vi "Path_Test2020_TankRobot_ScanIndex_CreateFile.vi"() -> ()   [LabVIEW 2019]
uses:
  Pathfinder-Lib/VIs/Waypoint.ctl
  <vilib>/Rock Robotics/WPI/DriverStation/WPI_DriverStationRobotMode2.ctl
  Pathfinder-Lib/VIs/Wheel_Ctrl_Path_Element.ctl
  Pathfinder-Lib/VIs/Wheel_Ctrl_Path.ctl
  Pathfinder-Lib/Pathfinder.lvlib
  Robot Global Data.vi
  <vilib>/Rock Robotics/SystemInterfaces/AI/FPGA_AIGyroChannel.ctl
  <vilib>/Rock Robotics/Network Tables/NT Write Number.vi
  <vilib>/Rock Robotics/WPI/Counter/WPI_CounterDigitalInputToDigitalSource.vi
  <vilib>/Rock Robotics/SystemInterfaces/DIO/FPGA_DIOChannel.ctl
  <vilib>/Rock Robotics/WPI/Encoder/WPI_EncoderType.ctl
  <vilib>/Rock Robotics/Network Tables/NT Write Numeric Array.vi
  <vilib>/addons/control/pid/NI_PID_pid.lvlib
  <vilib>/Rock Robotics/SystemInterfaces/DIO/FPGA_DIOPWMChannel.ctl
  <vilib>/Rock Robotics/WPI/SafetyOutput/WPI_SafetyOutputConfigMenu.ctl
  Secret_Control_Library_Protected/Secret_Control_Library_Protected.lvlib
  <vilib>/addons/control/pid/pid.llb/PID (DBL).vi
  <vilib>/Rock Robotics/WPI/Gyro/WPI_GyroAnalogOpen.vi
  <vilib>/Rock Robotics/WPI/RobotDrive/WPI_RobotDriveOpen2MotorWithTalon.vi
panel:
  in  "Tab Control 3":enum32{"Robot Data", "Path Definition"}(tab)
  in  "Real max\n speed":dbl=84.0
  in  "wheelbase_width":dbl=20.866
  in  "max_jerk":dbl=120.0
  in  "max_acceleration":dbl=65.0
  in  "max_velocity":dbl=70.0
  in  "?":T1[](array[typedef])=[{"x"=15.0, "y"=105.0, "angle"=0.0}, {"x"=35.0, "y"=105.0, "angle"=0.0}, {"x"=210.0, "y"=32.0, "angle"=0.0}, {"x"=230.0, "y"=32.0, "angle"=0.0}, {"x"=455.0, "y"=32.0, "angle"=0.0}, {"x"=625.0, "y"=98.0, "angle"=0.0}]
  in  "Path Results\ndT":dbl=0.02 format="%7.3f"
  in  "sample_count":i32=100000
  out "Path calculation error":errorcluster
  in  "Calculate\nPath":bool
  out "Complete,\nReady to \nExecute":bool
  out "Path \nSpeed > \nMax":bool
  in  "Rev\nDirection":bool
  in  "Tab Control 2":enum32{"Create File", "Robot Execution"}(tab)
  in  "Include Step":bool=TRUE
  in  "End Path CMD":i32=64
  in  "Cont Path CMD":i32=62
  in  "Start Path CMD":i32=60
  in  "Starting Step":i32
  in  "Command List Path Comment":string
  in  "Command List File Name":path
  in  "CreateCmdList":bool
  in  "Ramsete ?":bool=TRUE
  out "Robot Mode":T2
  out "Distance Error":dbl[](array[numeric]) format="%14.2f"
  out "Heading Error":dbl format="%14.2f"
  in  "Use Gyro\nCompensation":bool=TRUE
  out "Distance":dbl[](array[numeric]) format="%19.2f"
  in  "Gyro Comp PID gains":T3={"proportional gain (Kc)"=0.065, "integral time (Ti, min)"=0.004, "derivative time (Td, min)"=0.0} {"derivative time (Td, min)" format="%.4f"; "integral time (Ti, min)" format="%.4f"; "proportional gain (Kc)" format="%.4f"}
  out "Heading":dbl format="%18.2f"
  out "Gyro Comp":dbl format="%18.2f"
  out "Heading Demand":dbl format="%18.2f"
  in  "Execute\nPath":bool
  out "Robot\nExecuting":bool
  out "Path Distance":dbl[](array[numeric]) format="%19.2f"
  in  "Stop\nProgram":bool
  in  "Tab Control":T4(tab)
  out "Position":cluster{dbl[], dbl[]}[](graph)
  out "Path":T5(graph)
  out "Size":i32
  out "Robot Path Data":T6[](array[typedef]) {"D Time" format="%13.3f"; "Angle" format="%13.3f"; "R dist" format="%13.3f"; "L dist" format="%13.3f"; "R spd" format="%13.3f"; "L spd" format="%13.3f"; "T Time" format="%13.3f"}
  out "Wheel dmd":T7(graph)
  out "Gyro Cht":cluster{"GyroContinuous":dbl, "Angle":dbl}(graph)
  out "Err Chart":cluster{dbl, dbl, dbl}(graph)
  # "ROBOT DATA"
  # "INCHES/SEC"
  # "INCHES/SEC"
  # "INCHES/SEC^2"
  # "?? INCHES/SEC^3"
  # "Simulated robot is 20.866"
  # "INCHES"
  # "PATH DEFINITION"
  # "SEC"
  # "ROBOT EXECUTION\n(disabled...)"
  # "Instructions:\nThis should create a path, show the data on the various tabs and optionally write the motor demands and expected results to a file for use on a a robot..\n1) Enter robot data on Robot Data Tab\n2) Define your path definitions.\n3) Define the time increment.  0.020 is chosen since that matches the normal loop time.\n4) Press calculate path.  If a good path was calculated it will be displayed on the Tank Data tab, and the Ready to Execute will indicate execution can begin.\nThe path can be recalculated many times before selecting execute.\n\nTo write to a file.\n5) Select the file name\n6) This example uses \"steps\", sequential numbers for inclusion into a list based autonomous routine.  Including the step number if optional.\n7) This uses command numbers to indicate first, last, and intermediate steps.  This allows some simplification of the execution routine.  It\nalso allows the path to be executed backwards if desired.  The command numbers are changeable.\n8) Press \"Create Command List\".\n\nNotes:\n- PC robot simulataion is disabled in this program.  The code is still there if you want to restore it and try it out.  Use one of the other test programs \nto simulate the path on a PC.\n- The path generation logic doesn't account distribution of speed to the left and right wheels.  As a result the maximum speed can be exceeded.\nIf this happens, but Path Speed > Max light will light and Ready to Execute will not light.  Lower the maximum speed in the Robot Data tab\nand recalulate the path.\n- 2019 playing field size - width: 26 ft 11.25 In = 323.25 in , length: 52 ft 5.25 in = 629.25 in  (I didn't verify this for the 2020 version.)"
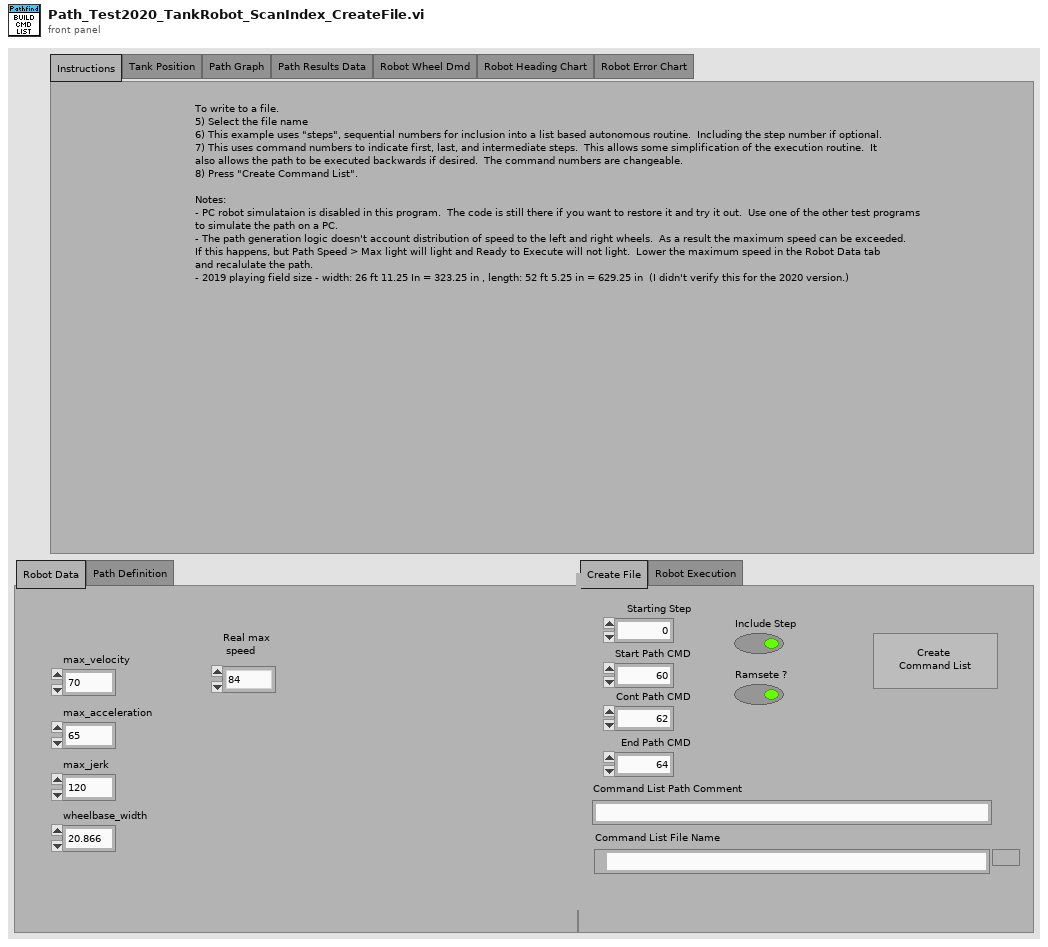
[diagram p1: front panel]
types:
  T1 = typedef "Pathfinder.lvlib/Waypoint.ctl" = cluster{"x":dbl, "y":dbl, "angle":dbl}
  T2 = typedef "WPI_DriverStationRobotMode2.ctl" = enum16{"Autonomous Disabled", "Autonomous Enabled", "Teleop Disabled", "Teleop Enabled", "Disconnected", "Finish", "Test Disabled", "Test Enabled", "Emergency Stopped"}
  T3 = cluster{"proportional gain (Kc)":dbl, "integral time (Ti, min)":dbl, "derivative time (Td, min)":dbl}
  T4 = enum32{"Instructions", "Tank Position", "Path Graph", "Path Results Data", "Robot Wheel Dmd", "Robot Heading Chart", "Robot Error Chart"}
  T5 = cluster{"position":dbl, "velocity":dbl, "acceleration":dbl, "jerk":dbl, "heading":dbl}[]
  T6 = typedef "Pathfinder.lvlib/Wheel_Ctrl_Path_Element.ctl" = cluster{"T Time":dbl, "L spd":dbl, "R spd":dbl, "L dist":dbl, "R dist":dbl, "Angle":dbl, "D Time":dbl}
  T7 = cluster{"Output":dbl, "Output":dbl, "output":dbl}
  T8 = typedef "Pathfinder.lvlib/Wheel_Ctrl_Path.ctl" = cluster{"Wheel_Ctrl_Elements":T6[], "NumberOfElements":u32, "DeltaMillseconds":i32}
  T9 = typedef "Pathfinder.lvlib/Segment.ctl" = cluster{"dt":dbl, "x":dbl, "y":dbl, "position":dbl, "velocity":dbl, "acceleration":dbl, "jerk":dbl, "heading":dbl}
  T10 = cluster{"position":dbl, "velocity":dbl, "acceleration":dbl, "jerk":dbl, "heading":dbl}
  T11 = typedef "WPI_SafetyOutputConfigMenu.ctl" = enum16{"Enable", "Disable"}
  T12 = typedef "WPI_EncoderType.ctl" = enum16{"1x", "2x", "4x"}
  T13 = typedef "FPGA_AIGyroChannel.ctl" = enum8{"AI 0", "AI 1", "Invalid"}
  T14 = enum32{"Instructions", "Robot Data", "Tank Position", "Path Graph", "Path Results Data", "Robot Wheel Dmd", "Robot Heading Chart", "Robot Error Chart"}
  T15 = typedef "FPGA_DIOPWMChannel.ctl" = enum8{"PWM 0", "PWM 1", "PWM 2", "PWM 3", "PWM 4", "PWM 5", "PWM 6", "PWM 7", "PWM 8", "PWM 9", "PWM MXP 0", "PWM MXP 1", "PWM MXP 2", "PWM MXP 3", "PWM MXP 4", "PWM MXP 5", "PWM MXP 6", "PWM MXP 7", "PWM MXP 8", "PWM MXP 9", "Invalid"}
  T16 = typedef "FPGA_DIOChannel.ctl" = enum8{"DIO 0", "DIO 1", "DIO 2", "DIO 3", "DIO 4", "DIO 5", "DIO 6", "DIO 7", "DIO 8", "DIO 9", "DIO MXP 0", "DIO MXP 1", "DIO MXP 2", "DIO MXP 3", "DIO MXP 4", "DIO MXP 5", "DIO MXP 6", "DIO MXP 7", "DIO MXP 8", "DIO MXP 9", "DIO MXP 10", "DIO MXP 11", "DIO MXP 12", "DIO MXP 13", "DIO MXP 14", "DIO MXP 15", "SPI Port CS1", "SPI Port CS2", "SPI Port CS3", "SPI Port MISO", "SPI Port MOSI", "Invalid"}
  T17 = typedef "WPI_RobotDriveDevRef.ctl" = cluster{"DevStatus":errorcluster, "Motors[]":T18[], "Square Inputs":bool, "Max Output":dbl}
  T18 = typedef "WPI_MotorControlDeviceRef.ctl" = cluster{"DeviceStatus":errorcluster, "Type":T19, "PWM":cluster{"PWM Channel":T15, "DeadBand":T20}, "CAN":cluster{"Device Number":u8, "SetOutput VI Ref":variant, "GetOutput VI Ref":variant, "Enable VI Ref":variant, "Disable VI Ref":variant, "Data":variant}, "Invert":bool, "DIO PWM":cluster{"PWM \"Enable\" Channel":T15, "DIOChannel":T16, "PWM Rate":dbl}}
  T19 = typedef "WPI_MotorControlType.ctl" = enum16{"PWM", "CAN", "DIO PWM"}
  T20 = typedef "WPI_PWMDeadband.ctl" = cluster{"Name":string, "maxPositivePwm":i32, "minPositivePwm":i32, "centerPwm":i32, "maxNegativePwm":i32, "minNegativePwm":i32, "angularRange":u16}
  T21 = typedef "WPI_DigitalInputDevRef.ctl" = cluster{"DevStatus":errorcluster, "DIO Channel":T16}
  T22 = typedef "FPGA_CounterEncoderSourceConvertionLVSourceType.ctl" = cluster{"DevStatus":errorcluster, "AnalogTriggerMode?":bool, "DigitalMode":cluster{"DIO Channel":T23}, "AnalogTriggerMode":cluster{"AnalogTriggerIndex":T24, "OutputType":T25}}
  T23 = typedef "FPGA_DIODigitalSourceChannel.ctl" = enum8{"DIO 0", "DIO 1", "DIO 2", "DIO 3", "DIO 4", "DIO 5", "DIO 6", "DIO 7", "DIO 8", "DIO 9", "DIO MXP 0", "DIO MXP 1", "DIO MXP 2", "DIO MXP 3", "DIO MXP 4", "DIO MXP 5", "DIO MXP 6", "DIO MXP 7", "DIO MXP 8", "DIO MXP 9", "DIO MXP 10", "DIO MXP 11", "DIO MXP 12", "DIO MXP 13", "DIO MXP 14", "DIO MXP 15", "SPI Port CS1", "SPI Port CS2", "SPI Port CS3", "SPI Port MISO", "SPI Port MOSI", "Disabled"}
  T24 = typedef "FPGA_AnalogTriggerIndex.ctl" = enum8{"Trig 0", "Trig 1", "Trig 2", "Trig 3", "Trig 4", "Trig 5", "Trig 6", "Trig 7", "Invalid"}
  T25 = typedef "FPGA_AnalogTriggerOutType.ctl" = enum16{"InWindow", "TriggerState", "Rising", "Falling"}
  T26 = typedef "WPI_EncoderDevRef.ctl" = cluster{"DevStatus":errorcluster, "EncoderIndex":T27, "CounterIndex":T28, "DistancePerCount":dbl, "Decoding Type":T12}
  T27 = typedef "FPGA_EncoderIdx.ctl" = enum8{"Enc 0", "Enc 1", "Enc 2", "Enc 3", "Enc 4", "Enc 5", "Enc 6", "Enc 7", "Invalid"}
  T28 = typedef "FPGA_CounterCtrSystemIndex.ctl" = enum8{"Ctr 0", "Ctr 1", "Ctr 2", "Ctr 3", "Ctr 4", "Ctr 5", "Ctr 6", "Ctr 7", "Invalid"}
  T29 = typedef "WPI_GyroDevRef.ctl" = cluster{"DevStatus":errorcluster, "Analog Channel":T30, "Gain (VoltsPerDegree/Second)":dbl, "Gyro Type":enum16{"Analog", "XRS450"}, "Handle":i32, "SPI Bus":T31, "Device Found":bool, "Sample Rate":dbl, "Calibrate On Open":bool, "Offset":dbl}
  T30 = typedef "FPGA_AIChannel.ctl" = enum8{"AI 0", "AI 1", "AI 2", "AI 3", "AI MXP 0", "AI MXP 1", "AI MXP 2", "AI MXP 3", "Invalid"}
  T31 = typedef "spi_bus.ctl" = enum16{"SPI On-Board, CS0", "SPI On-Board, CS1", "SPI On-Board, CS2", "SPI On-Board, CS3", "SPI MXP", "Invalid"}
  T32 = cluster{"GyroContinuous":dbl, "GyroContinuous":dbl}
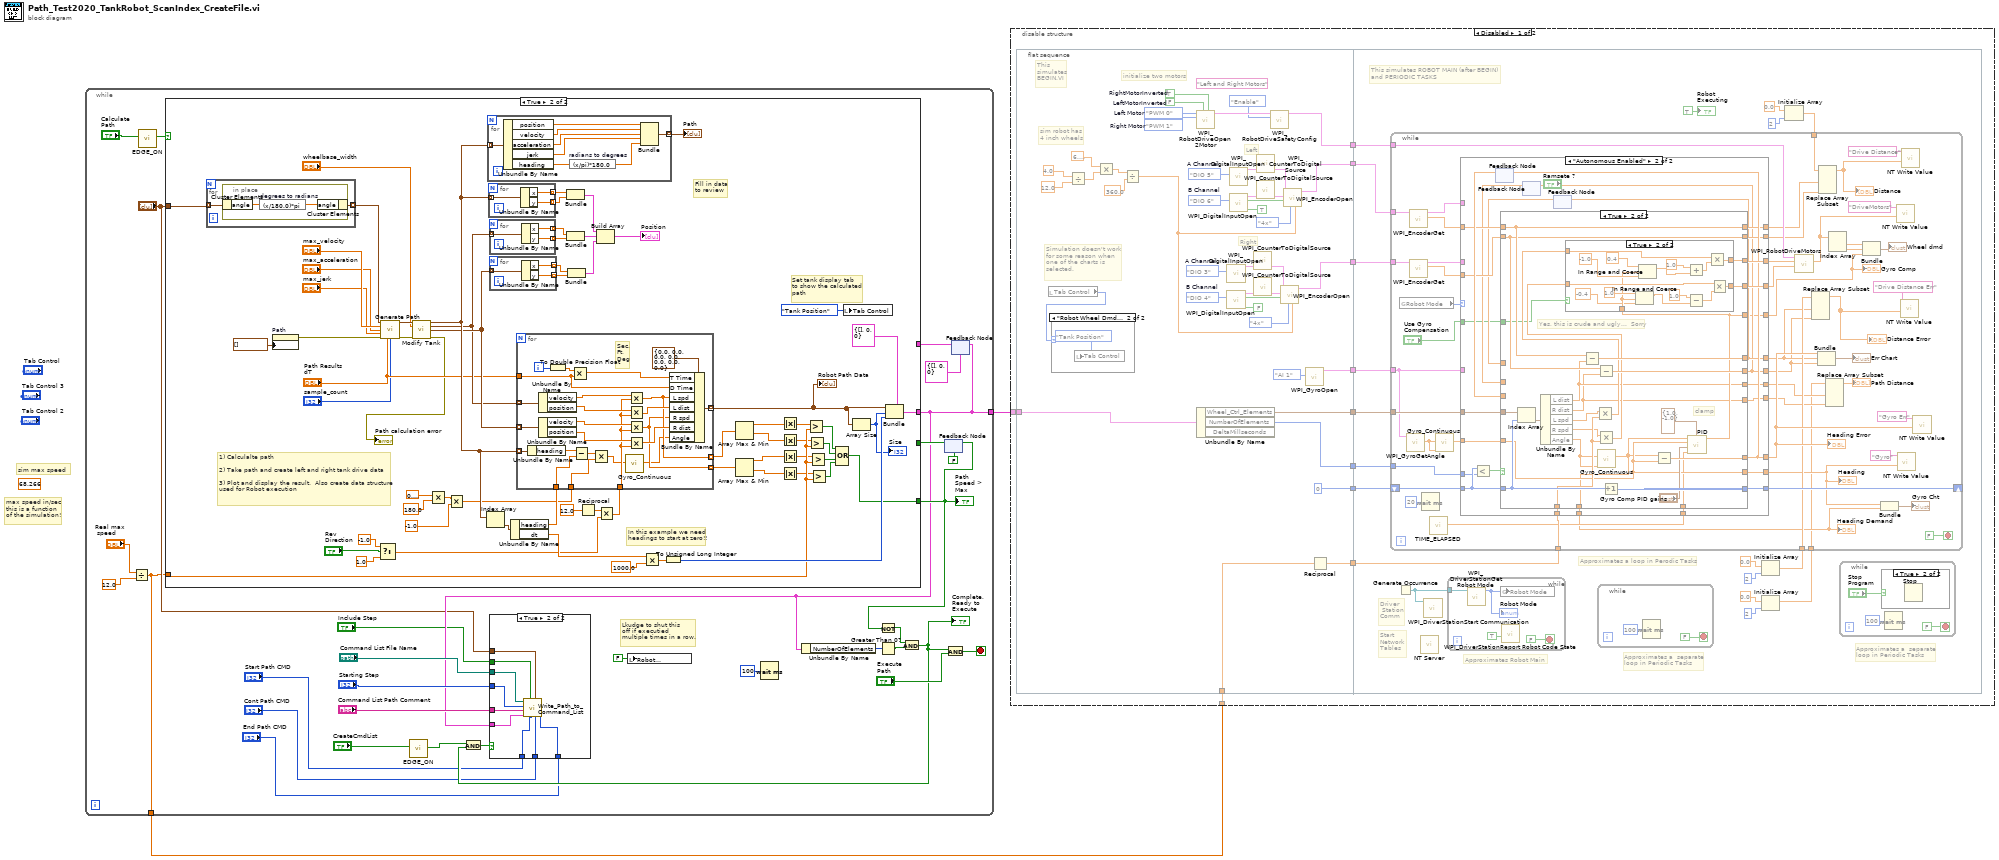
[diagram p0: block diagram]
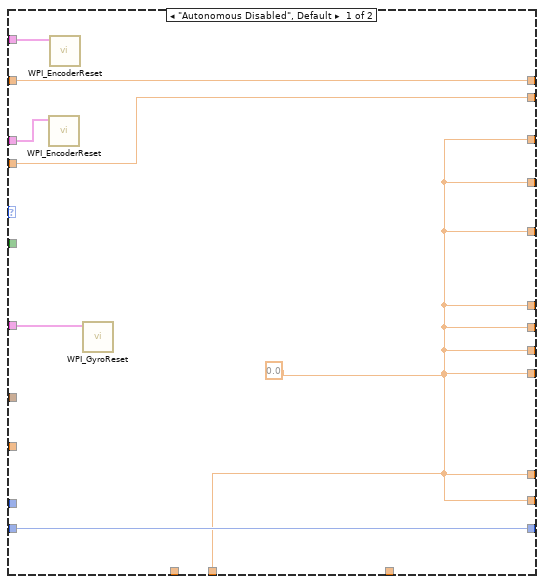
[diagram p4: hidden frame]
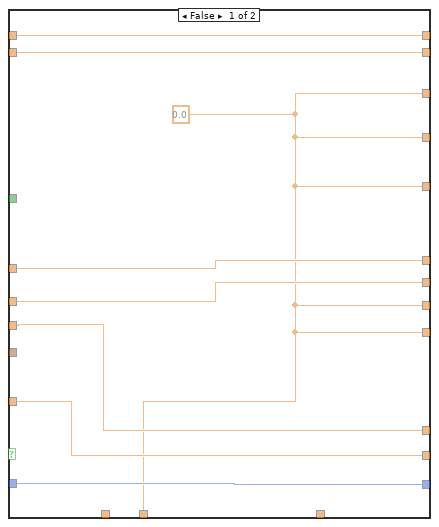
[diagram p5: hidden frame]
diagram:
  (unwired) 68.266 ("x")
  # "sim max speed"
  # "max speed in/sec\nthis is a function\nof the simulation!"
  n1 = while {
    tunnel: [w11] -> w2
    tunnel: [w3] -> w1
    stop <- w25 stop-if-true
    # "Lkudge to shut this\noff if executied\nmultiple times in a row."
    n2 = Divide(x="Real max\n speed", y=12.0) -> (x/y=w3:dbl)
    n3 = call "EDGE_ON.vi"("INPUT"="Calculate\nPath") -> ("EDGE ON"=w30:bool)  [unwired: 10 in]
    n4 = call "EDGE_ON.vi"("INPUT"="CreateCmdList") -> ("EDGE ON"=w13:bool)  [unwired: 10 in]
    n5 = local write "Robot\nExecuting"(FALSE ("Robot\nExecuting")) -> ()
    n6 = Wait (ms)(milliseconds to wait=u32 100) -> ()  [unwired: 1 out]
    n7 = feedback #1(FALSE) -> (w22:bool)
    n8 = feedback #2(T8 {"Wheel_Ctrl_Elements"=[], "NumberOfElements"=0, "DeltaMillseconds"=0} ("Wheel_Ctrl_Elements")) -> (w28:T8)
    n9 = case shown="True" w30 {
      tunnel: [w43 w71] -> w11
      tunnel: w28 -> [w43 _]
      tunnel: w3 -> [_ w69]
      tunnel: [w42 w60] -> w19
      tunnel: w22 -> [w42 _]
      tunnel: "?" -> [_ w50]
      frame False {
      }
      frame True {
        # "Set tank display tab\nto show the calculated\npath"
        # "Fill in data\nto review"
        # "1) Calculalte path\n\n2) Take path and create left and right tank drive data\n\n3) Plot and display the result.  Also create data structure\nused for Robot execution"
        # "In this example we need\nheadings to start at zero!!"
        n10 = for {
          tunnel: w50 -> [w135] mode=indexing
          tunnel: [w134] -> w97 mode=indexing
          n11 = in-place {
            n12 = in-place-cluster #3(w135) -> ("angle"=w137:dbl)
            n13 = expression code="(x/180.0)*pi" "degrees to radians"(w137) -> (w136:dbl)
            n14 = in-place-cluster #3("angle"=w136) -> (w134:T1)
          }
        }
        n15 = property on="Path" class="WFChart (strict)"("History Data"=T5 []) -> (error out=w98:errorcluster)  [unwired: 2 in, 1 out]
        n16 = Select(t=-1.0, s="Rev\nDirection", f=1.0) -> (s? t:f=w44:dbl)
        n17 = call "Generate Path.vi"("path"=w97, "max_velocity"="max_velocity", "max_acceleration"="max_acceleration", "max_jerk"="max_jerk", "error in"=w98, "dt (.001)"="Path Results\ndT", "sample_count (100000)"="sample_count") -> ("Segments"=w99:T9[], "error out"=w86:errorcluster)  [unwired: 7 in]
        n18 = call "Modify Tank.vi"("Original"=w99, "wheelbase_width"="wheelbase_width", "error in"=w86) -> ("original"=w107:T9[], "left"=w103:T9[], "right"=w104:T9[], "error out"=→"Path calculation error":errorcluster)  [unwired: 9 in]
        n19 = Multiply(x=0.3183098861837907, y=180.0) -> (x*y=w106:dbl)
        n20 = Multiply(x=w106, y=-1.0) -> (x*y=w52:dbl)
        n21 = Index Array(array=w107) -> (element=w108:T9)  [unwired: 1 in]
        n22 = for {
          tunnel: w107 -> [w154] mode=indexing
          tunnel: [w148] -> w101 mode=indexing
          n23 = Unbundle By Name(w154) -> ("position"=w153:dbl, "velocity"=w152:dbl, "acceleration"=w151:dbl, "jerk"=w150:dbl, "heading"=w149:dbl)
          n24 = expression code="(x/pi)*180.0" "radians to degrees"(w149) -> (w147:dbl)
          n25 = Bundle("position"=w153, "velocity"=w152, "acceleration"=w151, "jerk"=w150, "heading"=w147) -> (w148:T10)  [unwired: 1 in]
        }
        "Path" <- w101
        n26 = for {
          tunnel: w107 -> [w140] mode=indexing
          tunnel: [w139] -> w94 mode=indexing
          tunnel: [w138] -> w95 mode=indexing
          n27 = Unbundle By Name(w140) -> ("x"=w139:dbl, "y"=w138:dbl)
        }
        n28 = for {
          tunnel: w103 -> [w146] mode=indexing
          tunnel: [w145] -> w88 mode=indexing
          tunnel: [w144] -> w89 mode=indexing
          n29 = Unbundle By Name(w146) -> ("x"=w145:dbl, "y"=w144:dbl)
        }
        n30 = for {
          tunnel: w104 -> [w143] mode=indexing
          tunnel: [w142] -> w90 mode=indexing
          tunnel: [w141] -> w91 mode=indexing
          n31 = Unbundle By Name(w143) -> ("x"=w142:dbl, "y"=w141:dbl)
        }
        n32 = Unbundle By Name(w108) -> ("heading"=w109:dbl, "dt"=w75:dbl)
        n33 = Bundle(w94, w95) -> (w96:cluster{dbl[], dbl[]})  [unwired: 1 in]
        n34 = Bundle(w88, w89) -> (w93:cluster{dbl[], dbl[]})  [unwired: 1 in]
        n35 = Bundle(w90, w91) -> (w92:cluster{dbl[], dbl[]})  [unwired: 1 in]
        n36 = Reciprocal(x=12.0) -> (1/x=w49:dbl)
        n37 = Build Array(w96, w93, w92) -> (→"Position":cluster{dbl[], dbl[]}[])
        n38 = Multiply(x=w49, y=w44) -> (x*y=w48:dbl)
        n39 = for {
          tunnel: "Path Results\ndT" -> [w129]
          tunnel: [w132] -> w59 mode=indexing
          tunnel: w48 -> [w124]
          tunnel: w103 -> [w121] mode=indexing
          tunnel: w104 -> [w120] mode=indexing
          tunnel: w107 -> [w119] mode=indexing
          tunnel: w109 -> [w112]
          tunnel: [w115] -> w58 mode=indexing
          tunnel: [w114] -> w57 mode=indexing
          tunnel: w52 -> [w113]
          i -> [w131]
          # "Sec,\nFt,\nDeg"
          n40 = Unbundle By Name(w119) -> ("heading"=w117:dbl)
          n41 = Unbundle By Name(w121) -> ("velocity"=w128:dbl, "position"=w127:dbl)
          n42 = Unbundle By Name(w120) -> ("velocity"=w126:dbl, "position"=w125:dbl)
          n43 = To Double Precision Float(number=w131) -> (double precision float=w133:dbl)
          n44 = Multiply(x=w133, y=w129) -> (x*y=w130:dbl)
          n45 = Subtract(x=w117, y=w112) -> (x-y=w118:dbl)
          n46 = Multiply(x=w118, y=w113) -> (x*y=w111:dbl)
          n47 = call "Gyro_Continuous.vi"("GyroInput"=w111) -> ("GyroContinuous"=w110:dbl)  [unwired: 10 in]
          n48 = Multiply(x=w128, y=w124) -> (x*y=w115:dbl)
          n49 = Multiply(x=w127, y=w124) -> (x*y=w123:dbl)
          n50 = Multiply(x=w126, y=w124) -> (x*y=w114:dbl)
          n51 = Multiply(x=w125, y=w124) -> (x*y=w122:dbl)
          n52 = Bundle By Name(cluster=T6 {"T Time"=0.0, "L spd"=0.0, "R spd"=0.0, "L dist"=0.0, "R dist"=0.0, "Angle"=0.0, "D Time"=0.0} ("Wheel dmd"), "T Time"=w130, "D Time"=w129, "L spd"=w115, "L dist"=w123, "R spd"=w114, "R dist"=w122, "Angle"=w110) -> (w132:T6)
        }
        "Robot Path Data" <- w59
        n53 = Multiply(x=w75, y=1000.0) -> (x*y=w73:dbl)
        n54 = To Unsigned Long Integer(number=w73) -> (unsigned 32bit integer=w72:u32)
        n55 = Array Max & Min(array=w58) -> (max value=w56:dbl, min value=w55:dbl)  [unwired: 2 out]
        n56 = Array Max & Min(array=w57) -> (max value=w54:dbl, min value=w53:dbl)  [unwired: 2 out]
        n57 = Absolute Value(x=w56) -> (abs(x)=w68:dbl)
        n58 = Absolute Value(x=w55) -> (abs(x)=w67:dbl)
        n59 = Absolute Value(x=w54) -> (abs(x)=w66:dbl)
        n60 = Absolute Value(x=w53) -> (abs(x)=w65:dbl)
        n61 = Greater?(x=w68, y=w69) -> (0:w64:bool)
        n62 = Greater?(x=w67, y=w69) -> (0:w63:bool)
        n63 = Greater?(x=w66, y=w69) -> (0:w62:bool)
        n64 = Greater?(x=w65, y=w69) -> (0:w61:bool)
        n65 = Compound Arithmetic op=OR(w64, w63, w62, w61) -> (w60:bool)
        n66 = local write "Tab Control"(T4."Tank Position" ("Tab Control")) -> ()
        n67 = Array Size(array=w59) -> (size(s)=w70:i32)
        "Size" <- w70
        n68 = Bundle(cluster=T8 {"Wheel_Ctrl_Elements"=[], "NumberOfElements"=0, "DeltaMillseconds"=0} ("Wheel_Ctrl_Elements"), "Wheel_Ctrl_Elements"=w59, "NumberOfElements"=w70, "DeltaMillseconds"=w72) -> (w71:T8)
      }
    }
    "Path \nSpeed > \nMax" <- w19
    n69 = Unbundle By Name(w11) -> ("NumberOfElements"=w27:u32)
    n70 = Not(x=w19) -> (.not. x?=w20:bool)
    n71 = Greater Than 0?(x=w27) -> (x > 0?=w21:bool)
    n72 = And(x=w20, y=w21) -> (x .and. y?=w12:bool)
    "Complete,\nReady to \nExecute" <- w12
    n73 = And(x=w13, y=w12) -> (x .and. y?=w14:bool)
    n74 = case shown="True" w14 {
      tunnel: "Command List File Name" -> [_ w41]
      tunnel: "Starting Step" -> [_ w40]
      tunnel: "Command List Path Comment" -> [_ w39]
      tunnel: w11 -> [_ w38]
      tunnel: "End Path CMD" -> [_ w37]
      tunnel: "Cont Path CMD" -> [_ w36]
      tunnel: "Start Path CMD" -> [_ w35]
      tunnel: "Include Step" -> [_ w34]
      tunnel: "?" -> [_ w33]
      frame False {
      }
      frame True {
        n75 = call "Write_Path_to_Command_List.vi"("LastCmdNumb"=w37, "CmdNumb"=w36, "WayPoints"=w33, "FirstCmdNumb"=w35, "Include Step"=w34, "Wheel_Ctrl_Elements"=w38, "Comment"=w39, "starting step"=w40, "Cmd List File"=w41) -> ()  [unwired: 3 in]
      }
    }
    n76 = feedback-in #1(w19) -> ()
    n77 = And(x=w12, y="Execute\nPath") -> (x .and. y?=w25:bool)
    n78 = feedback-in #2(w11) -> ()
  }
  n79 = disable-structure shown="Disabled" {
    disable-tunnel: w1 -> [w156 _]
    disable-tunnel: w2 -> [w155 _]
    frame Disabled {
      n80 = flat-sequence {
        tunnel: w155 -> [w171]
        tunnel: [w174] -> w164
        tunnel: [w204] -> w163
        tunnel: [w172] -> w162
        tunnel: [w173] -> w161
        tunnel: [w170] -> w160
        tunnel: [w169] -> w159
        tunnel: [w168] -> w158
        tunnel: w156 -> [w167]
        tunnel: [0] -> w157
        tunnel: w164 -> [w223]
        tunnel: w163 -> [w222]
        tunnel: w162 -> [w221]
        tunnel: w161 -> [w214]
        tunnel: w160 -> [w224]
        tunnel: w159 -> [w213]
        tunnel: w158 -> [w208]
        tunnel: w157 -> [w207]
        frame #0 {
          w188 = FPGA_DIOPWMChannel."PWM 1"  # Right Motor
          w187 = FPGA_DIOPWMChannel."PWM 0"  # Left Motor
          (unwired) "Left and Right Motors" ("refnum name")
          w189 = FALSE  # LeftMotorInverted
          w190 = TRUE  # RightMotorInverted
          w182 = FPGA_DIOChannel."DIO 4"  # B Channel
          w181 = FPGA_DIOChannel."DIO 3"  # A Channel
          w178 = FPGA_DIOChannel."DIO 6"  # B Channel
          w177 = FPGA_DIOChannel."DIO 5"  # A Channel
          # "Simulation doesn't work\nfor some reason when\none of the charts is\nselected."
          # "This \nsimulates\nBEGIN.VI"
          # "sim robot has\n4 inch wheels"
          # "initialize two motors"
          # "Right"
          # "Left"
          n81 = local read "Tab Control"() -> (w165:T4)
          n82 = case shown="\"Robot Wheel Dmd\"..\"Robot Error Chart\"" w165 {
            frame Default {
            }
            frame "Robot Wheel Dmd".."Robot Error Chart" {
              n83 = local write "Tab Control"(T14."Tank Position" ("Tab Control")) -> ()
            }
          }
          n84 = Divide(x=4.0, y=12.0) -> (x/y=w200:dbl)
          n85 = Multiply(x=6.283185307179586, y=w200) -> (x*y=w201:dbl)
          n86 = Divide(x=w201, y=360.0) -> (x/y=w202:dbl)
          n87 = call-poly <vilib>:"WPI_RobotDriveOpen2Motor.vi"("Right Motor Inverted"=w190, "Left Motor Inverted"=w189, "Right Motor"=w188, "Left Motor"=w187) -> ("RobotDriveDevRef"=w203:T17)  [unwired: 1 in, 6 out]
          n88 = Unbundle By Name(w171) -> ("Wheel_Ctrl_Elements"=w170:T6[], "NumberOfElements"=w169:u32)  [unwired: 1 out]
          n89 = call <vilib>:"WPI_DigitalInputOpen.vi"("DIO Channel"=w181) -> ("DigitalInputDevRef"=w198:T21)  [unwired: 1 in, 9 out]
          n90 = call <vilib>:"WPI_DigitalInputOpen.vi"("DIO Channel"=w182) -> ("DigitalInputDevRef"=w197:T21)  [unwired: 1 in, 9 out]
          n91 = call <vilib>:"WPI_DigitalInputOpen.vi"("DIO Channel"=w177) -> ("DigitalInputDevRef"=w194:T21)  [unwired: 1 in, 9 out]
          n92 = call <vilib>:"WPI_DigitalInputOpen.vi"("DIO Channel"=w178) -> ("DigitalInputDevRef"=w193:T21)  [unwired: 1 in, 9 out]
          n93 = call-poly <vilib>:"WPI_CounterToDigitalSource.vi"("DigitalInputDevRef"=w198) -> ("Digital Source"=w199:T22)  [unwired: 6 out]
          n94 = call-poly <vilib>:"WPI_CounterToDigitalSource.vi"("DigitalInputDevRef"=w197) -> ("Digital Source"=w196:T22)  [unwired: 6 out]
          n95 = call-poly <vilib>:"WPI_CounterToDigitalSource.vi"("DigitalInputDevRef"=w194) -> ("Digital Source"=w195:T22)  [unwired: 6 out]
          n96 = call-poly <vilib>:"WPI_CounterToDigitalSource.vi"("DigitalInputDevRef"=w193) -> ("Digital Source"=w192:T22)  [unwired: 6 out]
          n97 = call <vilib>:"WPI_RobotDriveSafetyConfig.vi"("mode"=WPI_SafetyOutputConfigMenu."Enable", "RobotDriveDevRef"=w203) -> ("RobotDriveDevRef"=w174:T17)  [unwired: 8 in, 1 out]
          n98 = call <vilib>:"WPI_EncoderOpen.vi"("DistancePerCount"=w202, "Decoding Type"=WPI_EncoderType."4x", "Invert Direction (False)"=FALSE, "BSource"=w196, "ASource"=w199) -> ("EncoderDevRef"=w173:T26)  [unwired: 3 in, 3 out]
          n99 = call <vilib>:"WPI_EncoderOpen.vi"("DistancePerCount"=w202, "Decoding Type"=WPI_EncoderType."4x", "Invert Direction (False)"=TRUE, "BSource"=w192, "ASource"=w195) -> ("EncoderDevRef"=w172:T26)  [unwired: 3 in, 3 out]
          n100 = call-poly <vilib>:"WPI_GyroOpen.vi"("Analog Channel"=FPGA_AIGyroChannel."AI 1") -> ("GyroDevRef"=w204:T29)  [unwired: 8 in, 2 out]
          n101 = Reciprocal(x=w167) -> (1/x=w168:dbl)
        }
        frame #1 {
          # "Approximates a  separate\nloop in Periodic Tasks"
          # "This simulates ROBOT MAIN (after BEGIN)\nand PERIODIC TASKS"
          # "Approximates a loop in Perodic Tasks"
          # "Approximates a  separate\nloop in Periodic Tasks"
          # "Approximates Robot Main"
          # "Start\nNetwork\nTables"
          # "Driver\n Station\nComm"
          n102 = Generate Occurrence() -> (w225:refnum<k4>)
          n103 = call <vilib>:"NT Server.vi"() -> ()  [unwired: 12 in]
          n104 = call <vilib>:"WPI_DriverStationStart Communication.vi"("occurrence"=w225) -> ()  [unwired: 11 in]
          n105 = while {
            tunnel: w225 -> [w367]
            stop <- FALSE stop-if-true
            n106 = call <vilib>:"WPI_DriverStationGet Robot Mode.vi"("DS Occurrence"=w367) -> ("Robot Mode"=w364:T2)  [unwired: 1 in, 9 out]
            "Robot Mode" <- w364
            n107 = global write "Robot Global Data.vi" "Robot Mode"(w364) -> ()
            n108 = call <vilib>:"WPI_DriverStationReport Robot Code State.vi"("TeleOp"=TRUE ("Autonomous")) -> ()  [unwired: 10 in, 1 out]
          }
          n109 = while {
            stop <- FALSE stop-if-true
            n110 = Wait (ms)(milliseconds to wait=u32 100) -> ()  [unwired: 1 out]
          }
          n111 = Initialize Array(0.0, 2 ("dimension size")) -> (w215:dbl[])
          n112 = Initialize Array(0.0, 2 ("dimension size")) -> (w209:dbl[])
          n113 = Initialize Array(0.0, 2 ("dimension size")) -> (w218:dbl[])
          n114 = while {
            tunnel: w224 -> [w270]
            tunnel: w223 -> [w275]
            shift-right: [w271] -> _
            shift-left: w207 -> [w272]
            tunnel: w222 -> [w267]
            tunnel: w221 -> [w265]
            tunnel: w208 -> [w259]
            tunnel: w218 -> [w255]
            tunnel: w215 -> [w251]
            tunnel: w214 -> [w235]
            tunnel: w213 -> [w234]
            tunnel: w209 -> [w230]
            stop <- FALSE stop-if-true
            n115 = global read "Robot Global Data.vi" "Robot Mode"() -> (w276:T2)
            n116 = call <vilib>:"WPI_GyroGetAngle.vi"("GyroDevRef"=w267) -> ("Angle"=w241:dbl)  [unwired: 7 in, 3 out]
            n117 = call <vilib>:"WPI_EncoderGet.vi"("EncoderDevRef"=w265) -> ("Distance"=w262:dbl, "EncoderDevRef"=w236:T26)  [unwired: 5 in, 4 out]
            n118 = call <vilib>:"WPI_EncoderGet.vi"("EncoderDevRef"=w235) -> ("Distance"=w261:dbl, "EncoderDevRef"=w264:T26)  [unwired: 5 in, 4 out]
            n119 = Wait (ms)(milliseconds to wait=u32 20) -> ()  [unwired: 1 out]
            n120 = call "TIME_ELAPSED.vi"() -> ("Elapsed Sec"=w240:dbl)  [unwired: 11 in]
            n121 = call "Gyro_Continuous.vi"("GyroInitial"=w241, "GyroInput"=w241) -> ("GyroContinuous"=w247:dbl)  [unwired: 9 in]
            n122 = case shown="\"Autonomous Enabled\"" w276 {
              tunnel: [w278 w307] -> w274
              tunnel: [w278 w308] -> w273
              tunnel: w272 -> [w284 w310]
              tunnel: [w284 w309] -> w271
              tunnel: w270 -> [_ w306]
              tunnel: w259 -> [_ w304]
              tunnel: w267 -> [w283 _]
              tunnel: w247 -> [_ w303]
              tunnel: [w278 w302] -> w238
              tunnel: [w278 w301] -> w257
              tunnel: w264 -> [w282 _]
              tunnel: w262 -> [w281 w299]
              tunnel: w261 -> [w280 w298]
              tunnel: [w281 w297] -> w254
              tunnel: [w280 w296] -> w253
              tunnel: [w278 w292] -> w248
              tunnel: [w278 w293] -> w249
              tunnel: "Use Gyro\nCompensation" -> [_ w291]
              tunnel: [w278 w290] -> w243
              tunnel: w240 -> [_ w289]
              tunnel: [w278 w288] -> w237
              tunnel: w236 -> [w279 _]
              tunnel: w234 -> [_ w287]
              tunnel: [w278 w286] -> w232
              tunnel: [w278 w285] -> w231
              frame "Autonomous Disabled", Default {
                w278 = 0.0
                n123 = call <vilib>:"WPI_EncoderReset.vi"("EncoderDevRef"=w282) -> ()  [unwired: 9 in, 2 out]
                n124 = call <vilib>:"WPI_EncoderReset.vi"("EncoderDevRef"=w279) -> ()  [unwired: 9 in, 2 out]
                n125 = call <vilib>:"WPI_GyroReset.vi"("GyroDevRef"=w283) -> ()  [unwired: 9 in, 2 out]
              }
              frame "Autonomous Enabled" {
                n126 = Less?(x=w310, y=w287) -> (x < y?=w305:bool)
                n127 = feedback #4() -> (w300:dbl)  [unwired: 1 in]
                n128 = feedback #5() -> (w294:dbl)  [unwired: 1 in]
                n129 = feedback #6() -> (w295:dbl)  [unwired: 1 in]
                n130 = case shown="True" w305 {
                  tunnel: w310 -> [w318 w343]
                  tunnel: [w318 w344] -> w309
                  tunnel: [w311 w341] -> w308
                  tunnel: [w311 w340] -> w307
                  tunnel: w306 -> [_ w324]
                  tunnel: w304 -> [_ w342]
                  tunnel: w303 -> [w317 w328]
                  tunnel: [w317 w328] -> w302
                  tunnel: [w316 w332] -> w301
                  tunnel: w300 -> [w316 _]
                  tunnel: w299 -> [w314 w339]
                  tunnel: [w314 w339] -> w297
                  tunnel: w298 -> [w315 w338]
                  tunnel: [w315 w338] -> w296
                  tunnel: w295 -> [w313 _]
                  tunnel: w294 -> [w312 _]
                  tunnel: [w312 w337] -> w292
                  tunnel: [w313 w336] -> w293
                  tunnel: w291 -> [_ w333]
                  tunnel: [w311 w329] -> w290
                  tunnel: w289 -> [_ w327]
                  tunnel: [w311 w326] -> w288
                  tunnel: [w311 w320] -> w286
                  tunnel: [w311 w319] -> w285
                  frame False {
                    w311 = 0.0
                  }
                  frame True {
                    # "Yes, this is crude and ugly...  Sorry"
                    # "clamp"
                    n131 = Index Array(array=w324, index=w343) -> (element=w322:T6)
                    n132 = Unbundle By Name(w322) -> ("L dist"=w320:dbl, "R dist"=w319:dbl, "L spd"=w325:dbl, "R spd"=w321:dbl, "Angle"=w323:dbl)
                    n133 = Subtract(x=w339, y=w320) -> (x-y=w336:dbl)
                    n134 = Multiply(x=w325, y=w342) -> (x*y=w335:dbl)
                    n135 = Subtract(x=w338, y=w319) -> (x-y=w337:dbl)
                    n136 = Multiply(x=w321, y=w342) -> (x*y=w334:dbl)
                    n137 = call "Gyro_Continuous.vi"("GyroInitial"=w323, "GyroInput"=w323) -> ("GyroContinuous"=w326:dbl)  [unwired: 9 in]
                    n138 = Increment(x=w343) -> (x+1=w344:i32)
                    n139 = Subtract(x=w326, y=w328) -> (x-y=w332:dbl)
                    n140 = call-poly <vilib>:"PID.vi"("output range"=cluster{"output high":dbl, "output low":dbl} {"output high"=1.0, "output low"=-1.0}, "dt (s)"=w327, "PID gains"="Gyro Comp PID gains", "process variable"=w328, "setpoint"=w326) -> ("output"=w329:dbl)  [unwired: 5 in, 1 out]
                    n141 = case shown="True" w333 {
                      tunnel: [w345 w357] -> w341
                      tunnel: w335 -> [w346 w356]
                      tunnel: [w346 w355] -> w340
                      tunnel: w334 -> [w345 w354]
                      tunnel: w329 -> [_ w348]
                      frame False {
                      }
                      frame True {
                        n142 = In Range and Coerce(upper limit=1.0, x=w348, lower limit=-0.4 ("x")) -> (coerced(x)=w350:dbl)  [unwired: 1 out]
                        n143 = In Range and Coerce(upper limit=0.4, x=w348, lower limit=-1.0 ("x")) -> (coerced(x)=w351:dbl)  [unwired: 1 out]
                        n144 = Add(x=1.0, y=w351) -> (x+y=w360:dbl)
                        n145 = Subtract(x=1.0, y=w350) -> (x-y=w358:dbl)
                        n146 = Multiply(x=w356, y=w360) -> (x*y=w355:dbl)
                        n147 = Multiply(x=w354, y=w358) -> (x*y=w357:dbl)
                      }
                    }
                  }
                }
                n148 = feedback-in #4(w301) -> ()
                n149 = feedback-in #5(w292) -> ()
                n150 = feedback-in #6(w293) -> ()
              }
            }
            "Heading Error" <- w257
            "Heading" <- w238
            "Gyro Comp" <- w243
            "Heading Demand" <- w237
            n151 = call <vilib>:"WPI_RobotDriveMotors.vi"("RightSpeed"=w273, "LeftSpeed"=w274, "RobotDriveDevRef"=w275) -> ("Motor Values"=w246:dbl[])  [unwired: 6 in, 2 out]
            n152 = Replace Array Subset(array=w251, new element #1=w249, new element #2=w248) -> (w250:dbl[])  [unwired: 2 in]
            "Distance Error" <- w250
            n153 = Bundle(w257, w249, w248) -> (→"Err Chart":cluster{dbl, dbl, dbl})  [unwired: 1 in]
            n154 = Replace Array Subset(array=w255, new element #1=w254, new element #2=w253) -> (w252:dbl[])  [unwired: 2 in]
            "Distance" <- w252
            n155 = Replace Array Subset(array=w230, new element #1=w232, new element #2=w231) -> (→"Path Distance":dbl[])  [unwired: 2 in]
            n156 = Index Array(array=w246) -> (element #1=w244:dbl, element #2=w245:dbl)  [unwired: 2 in]
            n157 = Bundle("Output"=w244, "Output"=w245, "output"=w243) -> (→"Wheel dmd":T7)  [unwired: 1 in]
            n158 = Bundle("GyroContinuous"=w238, "GyroContinuous"=w237) -> (→"Gyro Cht":T32)  [unwired: 1 in]
            n159 = call-poly <vilib>:"NT Write Value.vi"("Numeric Array"=w246, "Name"="DriveMotors") -> ()  [unwired: 9 in, 1 out]
            n160 = call-poly <vilib>:"NT Write Value.vi"("Numeric"=w238, "Name"="Gyro") -> ()  [unwired: 9 in, 1 out]
            n161 = call-poly <vilib>:"NT Write Value.vi"("Numeric Array"=w250, "Name"="Drive Distance Err") -> ()  [unwired: 9 in, 1 out]
            n162 = call-poly <vilib>:"NT Write Value.vi"("Numeric Array"=w252, "Name"="Drive Distance") -> ()  [unwired: 9 in, 1 out]
            n163 = call-poly <vilib>:"NT Write Value.vi"("Numeric"=w257, "Name"="Gyro Err") -> ()  [unwired: 9 in, 1 out]
          }
          n164 = while {
            stop <- FALSE stop-if-true
            n165 = case shown="True" "Stop\nProgram" {
              frame False {
              }
              frame True {
                n166 = Stop() -> ()  [unwired: 1 in]
              }
            }
            n167 = Wait (ms)(milliseconds to wait=u32 100) -> ()  [unwired: 1 out]
          }
          "Robot\nExecuting" <- TRUE ("Robot\nExecuting")
        }
      }
    }
    frame Enabled {
    }
  }
